vi "Send Message.vi"(6 "priority":i32, 8 "error in (no error)":errorcluster, 9 "timeout ms (-1)":i32=-1, 10 "Message":refnum<class "Message.lvclass">, 11 "TCP Stream in":refnum<class "TCP Stream.lvclass">) -> (0 "error out":errorcluster, 3 "TCP Stream out":refnum<class "TCP Stream.lvclass">)   [LabVIEW 2020, in "TCP Stream.lvclass"]
uses:
  TCP Stream.lvclass
  Abstract Classes/Message Stream/Message Stream.lvclass
  Abstract Classes/Cipher/Cipher.lvclass
  Abstract Classes/Message Flattener/Message Flattener.lvclass
  <vilib>/ActorFramework/Message/Message.lvclass
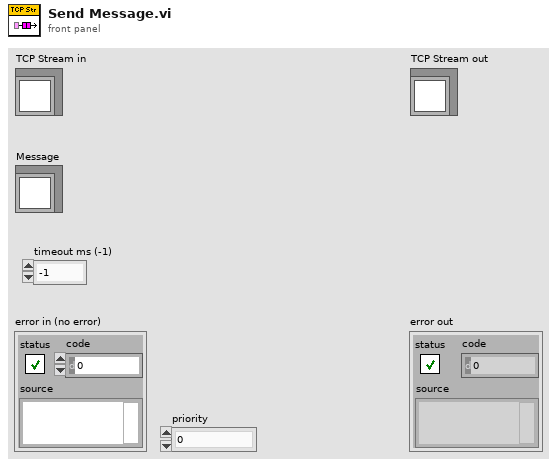
[diagram p1: front panel]
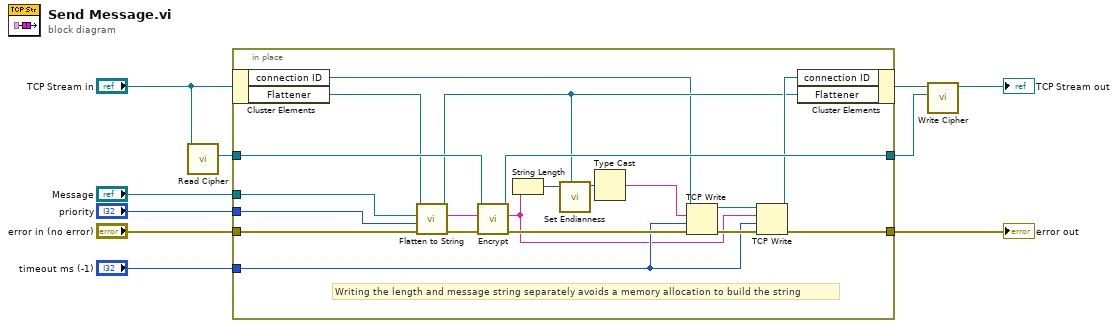
[diagram p0: block diagram]
diagram:
  n1 = call "Read Cipher.vi"("Message Stream in"="TCP Stream in") -> ("Cipher.lvclass"=w3:refnum<class "Cipher.lvclass">)  [unwired: 10 in]
  n2 = in-place {
    in-place-border: "error in (no error)" -> [w23]
    in-place-border: w3 -> [w28]
    in-place-border: [w27] -> w1
    in-place-border: "priority" -> [w22]
    in-place-border: "Message" -> [w21]
    in-place-border: "timeout ms (-1)" -> [w12]
    in-place-border: [w25] -> w5
    # "Writing the length and message string separately avoids a memory allocation to build the string"
    n3 = in-place-cluster #1("TCP Stream in") -> ("connection ID"=w15:refnum<k5>, "Flattener"=w20:refnum<class "Message Flattener.lvclass">)
    n4 = call-dynamic "Flatten to String.vi"("error in (no error)"=w23, "priority"=w22, "Message"=w21, "Flattener in"=w20) -> ("error out"=w24:errorcluster, "Flattened String"=w19:string, "Flattener out"=w17:refnum<class "Message Flattener.lvclass">)  [unwired: 5 in]
    n5 = call-dynamic "Encrypt.vi"("error in (no error)"=w24, "Plaintext"=w19, "Cipher in"=w28) -> ("error out"=w30:errorcluster, "Cyphertext"=w11:string, "Cipher out"=w27:refnum<class "Cipher.lvclass">)  [unwired: 6 in]
    n6 = String Length(string=w11) -> (length=w29:i32)
    n7 = call-dynamic "Set Endianness.vi"("Message Flattener in"=w17, "bytes to read"=w29) -> ("bytes to read"=w18:i32)  [unwired: 9 in]
    n8 = Type Cast(x=w18) -> (*(type *) &x=w13:string)  [unwired: 1 in]
    n9 = TCP Write(connection ID=w15, data in=w13, error in (no error)=w30, 9:w12) -> (connection ID out=w14:refnum<k5>, error out=w16:errorcluster)  [unwired: 1 out]
    n10 = TCP Write(connection ID=w14, data in=w11, error in (no error)=w16, 9:w12) -> (connection ID out=w26:refnum<k5>, error out=w25:errorcluster)  [unwired: 1 out]
    n11 = in-place-cluster #1("connection ID"=w26, "Flattener"=w17) -> (w2:refnum<class "TCP Stream.lvclass">)
  }
  "error out" <- w5
  n12 = call "Write Cipher.vi"("Cipher"=w1, "Message Stream in"=w2) -> ("Message Stream out"=→"TCP Stream out":refnum<class "TCP Stream.lvclass">)  [unwired: 9 in]
